vi "TankDriveHandler.vi"(6 "Sensitivity (.01)":dbl=0.01, 7 "Mode":T2=enum."Do", 8 "Error In (no error)":errorcluster, 9 "Right Motor Value (0)":dbl, 10 "Left Motor Value (0)":dbl, 11 "HalfSpeed (F)":bool) -> (0 "Error Out":errorcluster)   [LabVIEW 2012]
doc: "Handles input for tank drive. \nParameters:\n- Motor values: default to 0 if unwired.\n- Mode: Init or Do. Init will set the motors to 0 and prepare this VI for future calls, so this VI should be called with Init first. Do will update the motor values according to LeftMotorValue and RightMotorValue.\n- HalfSpeed: If true, cuts motor speed in half. Defaults to false.\n- Sensitivity: A measure of how big a change in joystick value is needed to trigger an event. Defaults to .01.\nIf the motor values changed significantly, a tank drive enstruction will be enqueued."
uses:
  State_Machine_Enum.ctl
  TankDriveInstruction.ctl
  QueueInstruction.ctl
  SubsystemEnum.ctl
  ActionEnum.ctl
  Robot Global Data.vi
panel:
  in  "TankDriveInstruction 2":T1
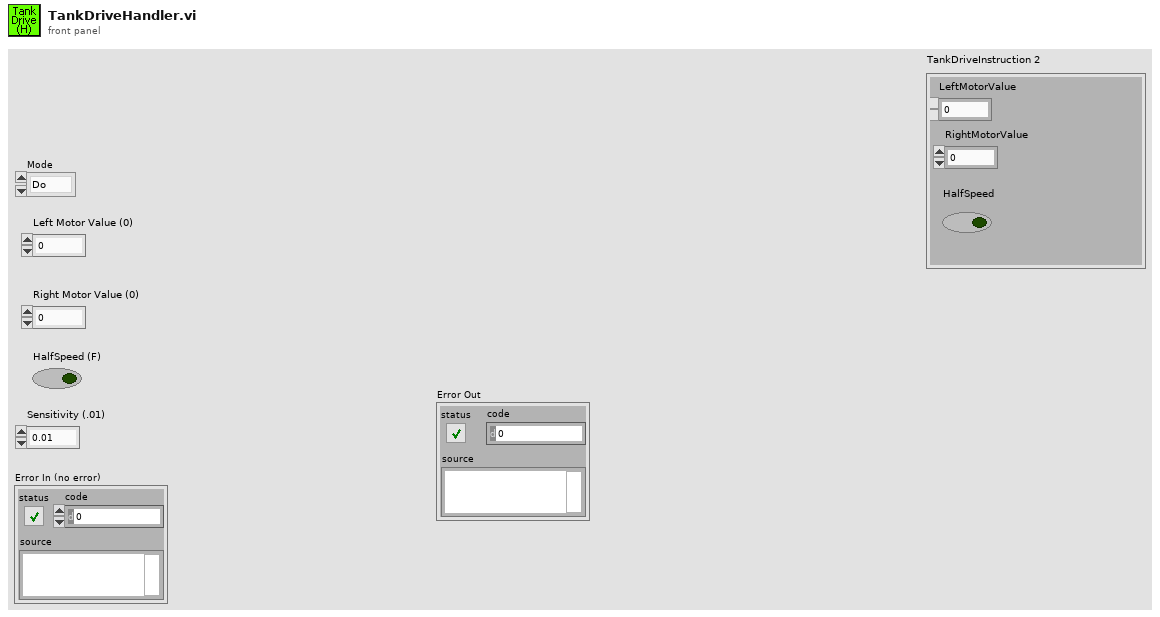
[diagram p1: front panel]
types:
  T1 = typedef "TankDriveInstruction.ctl" = cluster{"LeftMotorValue":dbl, "RightMotorValue":dbl, "HalfSpeed":bool}
  T2 = typedef "State_Machine_Enum.ctl" = enum16{"Idle", "Start", "Do", "Stop", "Init"}
  T3 = typedef "ActionEnum.ctl" = enum16{"Init", "SetValue"}
  T4 = typedef "SubsystemEnum.ctl" = enum16{"TankDrive", "FirePneumatic", "Climber", "ClimbWeight", "ShooterAngle"}
  T5 = typedef "QueueInstruction.ctl" = cluster{"Data":variant, "Subsystem":T4, "Action":T3}
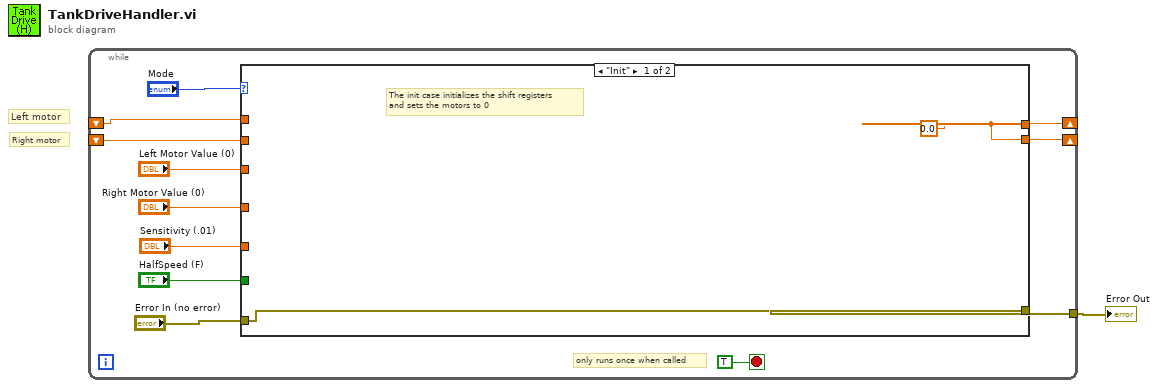
[diagram p0: block diagram]
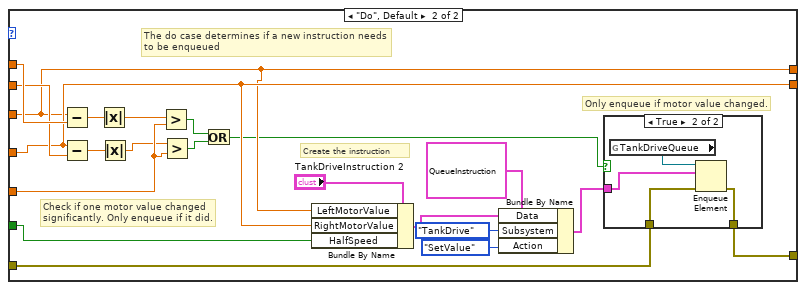
[diagram p2: hidden frame]
diagram:
  # "Right motor"
  # "Left motor"
  n1 = while {
    shift-right: [w9] -> _
    shift-left: _ -> [w7]
    shift-right: [w8] -> _
    shift-left: _ -> [w6]
    tunnel: [w5] -> w1
    stop <- TRUE stop-if-true
    # "only runs once when called"
    n2 = case shown="\"Init\"" "Mode" {
      tunnel: "Left Motor Value (0)" -> [_ w25]
      tunnel: "Right Motor Value (0)" -> [_ w26]
      tunnel: "Sensitivity (.01)" -> [_ w33]
      tunnel: "HalfSpeed (F)" -> [_ w24]
      tunnel: "Error In (no error)" -> [w15 w17]
      tunnel: [w14 w25] -> w9
      tunnel: [w14 w26] -> w8
      tunnel: w7 -> [_ w29]
      tunnel: w6 -> [_ w28]
      tunnel: [w15 w16] -> w5
      frame "Init" {
        w14 = 0.0
        # "The init case initializes the shift registers\nand sets the motors to 0"
      }
      frame "Do", Default {
        # "Only enqueue if motor value changed."
        # "Create the instruction"
        # "The do case determines if a new instruction needs\nto be enqueued"
        # "Check if one motor value changed\nsignificantly. Only enqueue if it did."
        n3 = Subtract(x=w25, y=w29) -> (x-y=w36:dbl)
        n4 = Subtract(x=w26, y=w28) -> (x-y=w35:dbl)
        n5 = Absolute Value(x=w36) -> (abs(x)=w34:dbl)
        n6 = Absolute Value(x=w35) -> (abs(x)=w32:dbl)
        n7 = Greater?(x=w34, y=w33) -> (0:w30:bool)
        n8 = Greater?(x=w32, y=w33) -> (0:w31:bool)
        n9 = Or(x=w30, y=w31) -> (x .or. y?=w19:bool)
        n10 = Bundle By Name(cluster="TankDriveInstruction 2", "LeftMotorValue"=w25, "RightMotorValue"=w26, "HalfSpeed"=w24) -> (w22:T1)
        n11 = Bundle By Name(cluster=T5 {"Data"=variant, "Subsystem"=enum."TankDrive", "Action"=enum."Init"} ("QueueInstruction"), "Data"=w22, "Subsystem"=SubsystemEnum."TankDrive", "Action"=ActionEnum."SetValue") -> (w18:T5)
        n12 = case shown="True" w19 {
          tunnel: w18 -> [_ w40]
          tunnel: w17 -> [w37 w39]
          tunnel: [w37 w38] -> w16
          frame False {
          }
          frame True {
            n13 = global read "Robot Global Data.vi" "TankDriveQueue"() -> (w41:refnum<queue>)
            n14 = Enqueue Element(queue=w41, element=w40, error in (no error)=w39) -> (error out=w38:errorcluster)  [unwired: 1 in, 2 out]
          }
        }
      }
    }
  }
  "Error Out" <- w1
